vi "read_ini_file.vi"(8 "error in (no error)":errorcluster, 11 "configuration file path":path=path "D:/config.ini") -> (0 "error out":errorcluster, 1 "values":string[](array[string]), 2 "keys":string[](array[string]), 3 "sections":string[](array[string]))   [LabVIEW 2022 SP3]
uses:
  <vilib>/Utility/config.llb/Read Key (String).vi
  <vilib>/Utility/config.llb/NI_LVConfig.lvlib
panel:
  out "element":string
  in  "index":i32
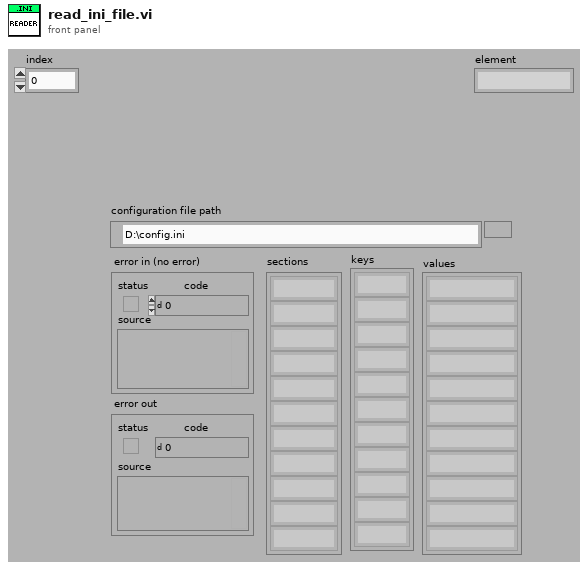
[diagram p1: front panel]
types:
  T1 = typedef "NI_LVConfig.lvlib/Config Data RefNum.ctl" = refnum<k1>
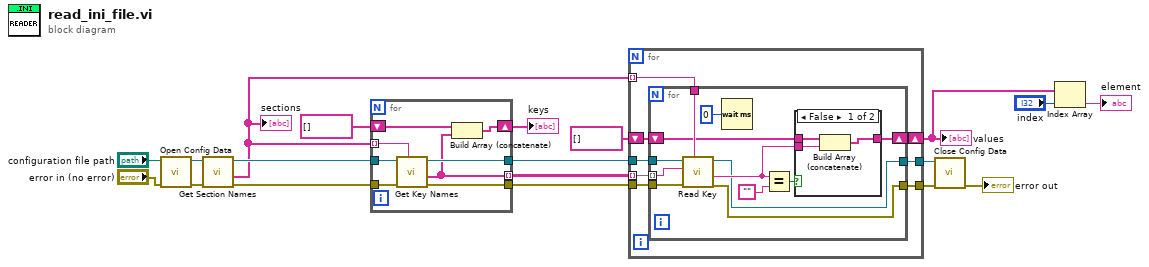
[diagram p0: block diagram]
diagram:
  n1 = call <vilib>:"Open Config Data.vi"("error in (no error)"="error in (no error)", "configuration file path"="configuration file path") -> ("error out"=w19:errorcluster, "refnum"=w18:T1)  [unwired: 7 in, 1 out]
  n2 = call <vilib>:"Get Section Names.vi"("error in (no error)"=w19, "refnum"=w18) -> ("error out"=w16:errorcluster, "section names"=w4:string[], "refnum out"=w17:T1)  [unwired: 7 in]
  "sections" <- w4
  n3 = for {
    tunnel: w17 -> [w27]
    tunnel: w16 -> [w26]
    tunnel: [w25] -> w11
    tunnel: [w24] -> w12
    tunnel: w4 -> [w23] mode=indexing
    shift-right: [w22] -> w5
    shift-left: string[] [] -> [w21]
    tunnel: [w20] -> w9 mode=indexing
    n4 = call <vilib>:"Get Key Names.vi"("section"=w23, "error in (no error)"=w26, "refnum"=w27) -> ("error out"=w25:errorcluster, "key names"=w20:string[], "refnum out"=w24:T1)  [unwired: 5 in, 1 out]
    n5 = Build Array (concatenate)(w21, w20) -> (w22:string[])
  }
  "keys" <- w5
  n6 = for {
    tunnel: w12 -> [w34]
    tunnel: w11 -> [w35]
    tunnel: w4 -> [w33] mode=indexing
    tunnel: w9 -> [w32] mode=indexing
    shift-right: [w31] -> w2
    shift-left: string[] [] -> [w30]
    tunnel: [w29] -> w7
    tunnel: [w28] -> w6
    n7 = for {
      tunnel: w34 -> [w45]
      tunnel: w33 -> [w47]
      tunnel: w32 -> [w44] mode=indexing
      tunnel: w35 -> [w43]
      shift-right: [w39] -> w31
      shift-left: w30 -> [w38]
      tunnel: [w36] -> w29
      tunnel: [w37] -> w28
      n8 = call-poly <vilib>:"Read Key.vi"("section"=w47, "error in (no error)"=w43, "key"=w44, "refnum"=w45) -> ("error out"=w37:errorcluster, "value"=w40:string, "refnum out"=w36:T1)  [unwired: 4 in, 1 out]
      n9 = Wait (ms)(milliseconds to wait=u32 0) -> ()  [unwired: 1 out]
      n10 = Equal?(x=w40, y="") -> (x = y?=w41:bool)
      n11 = case shown="False" w41 {
        tunnel: w40 -> [w50 _]
        tunnel: [w49 w51] -> w39
        tunnel: w38 -> [w48 w51]
        frame False {
          n12 = Build Array (concatenate)(w48, w50) -> (w49:string[])
        }
        frame True {
        }
      }
    }
  }
  "values" <- w2
  n13 = call <vilib>:"Close Config Data.vi"("error in (no error)"=w6, "refnum"=w7) -> ("error out"=→"error out":errorcluster)  [unwired: 8 in, 1 out]
  n14 = Index Array(array=w2, index="index") -> (element=→"element":string)
